vi "Actor Receive.vi"(11 "Dev Actor in":refnum<class "Dev Actor.lvclass">) -> (0 "error out":errorcluster, 2 "Msg":refnum<class "Msg Strategy.lvclass">)   [LabVIEW 2021, in "Dev Actor.lvlib" / "Dev Actor.lvclass"]
uses:
  Dev Actor.lvclass
  LVCAM/LVCAM/Msg Strategy/Msg Strategy.lvclass
  Dev Actor.lvclass/Dev Actor.ctl
  LVCAM/LVCAM/Actor/Actor.lvclass
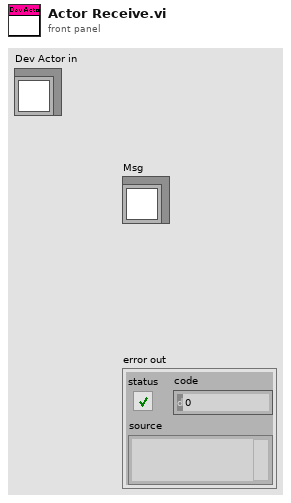
[diagram p1: front panel]
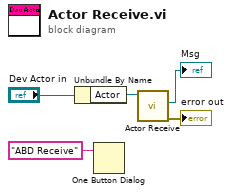
[diagram p0: block diagram]
diagram:
  n1 = Unbundle By Name("Dev Actor in") -> ("Actor"=w2:refnum<class "Actor.lvclass">)
  n2 = One Button Dialog(message="ABD Receive") -> ()  [unwired: 1 in, 1 out]
  n3 = call-dynamic "Actor Receive.vi"("Actor in"=w2) -> ("error out"=→"error out":errorcluster, "Msg"=→"Msg":refnum<class "Msg Strategy.lvclass">)  [unwired: 9 in]
